vi "SetTileByCode.vi"(8 "error in (no error)":errorcluster, 9 "Coordinates":T1, 10 "TileNumber":u16, 11 "Game in":refnum<class "Game.lvclass">) -> (0 "error out":errorcluster, 3 "Game out":refnum<class "Game.lvclass">)   [LabVIEW 2019, in "RT_Game.lvlib" / "Game.lvclass"]
uses:
  Game.lvclass
  Coordinate.ctl
  Game.lvclass/Game.ctl
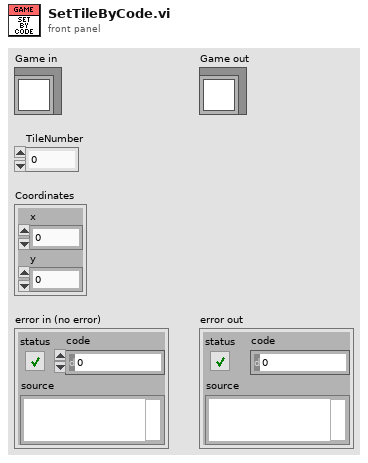
[diagram p1: front panel]
types:
  T1 = typedef "RT_Game.lvlib/Game.lvclass/Coordinate.ctl" = cluster{"x":dbl, "y":dbl}
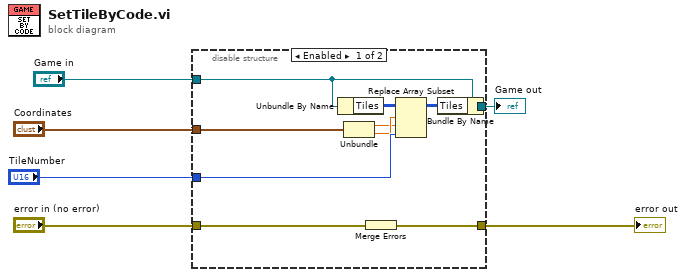
[diagram p0: block diagram]
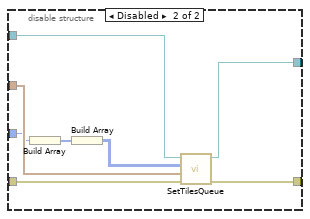
[diagram p2: hidden frame]
diagram:
  n1 = disable-structure shown="Enabled" {
    disable-tunnel: "Coordinates" -> [w16 w20]
    disable-tunnel: "TileNumber" -> [w15 w19]
    disable-tunnel: [w14 w21] -> w4
    disable-tunnel: "Game in" -> [w13 w22]
    disable-tunnel: "error in (no error)" -> [w8 w24]
    disable-tunnel: [w7 w23] -> w1
    frame Enabled {
      n2 = Unbundle By Name(w13) -> ("Tiles"=w9:u16[][])
      n3 = Unbundle(w16) -> ("x"=w11:dbl, "y"=w12:dbl)
      n4 = Merge Errors(w8) -> (w7:errorcluster)
      n5 = Replace Array Subset(array=w9, new element=w15, index (row)=w12, index (col)=w11) -> (w10:u16[][])
      n6 = Bundle By Name(cluster=w13, "Tiles"=w10) -> (w14:refnum<class "Game.lvclass">)
    }
    frame Disabled {
      n7 = Build Array(w19) -> (w18:u16[])
      n8 = Build Array(w18) -> (w17:u16[][])
      n9 = call "SetTilesQueue.vi"("error in (no error)"=w24, "Position"=w20, "TileCodes"=w17, "Game in"=w22) -> ("error out"=w23:errorcluster, "Game out"=w21:refnum<class "Game.lvclass">)  [unwired: 6 in]
    }
  }
  "error out" <- w1
  "Game out" <- w4
